vi "CH_LM App ResolutionMenu.vi"(4 "Action (query)":bool, 5 "error in":errorcluster, 6 "menubar":refnum<k9>, 7 "Menu String":string, 8 "Meter Index":i32) -> (0 "error out":errorcluster, 3 "Meter Index":i32)   [LabVIEW 2012, in "CH_LM App.lvlib"]
doc: "This VI is used to set/query the resolution of the displayed measurement value and check the corresponding menu items."
uses:
  CH_LM App.lvlib
  CH_LM.lvlib
  CH_LM/CH_LM Numeric Resolution.ctl
  CH_LM/CH_LM ProbeType.ctl
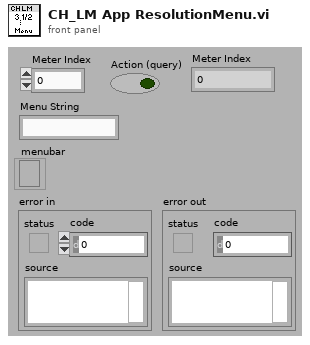
[diagram p1: front panel]
types:
  T1 = typedef "CH_LM.lvlib/CH_LM ProbeType.ctl" = enum16{"None", "Thermopile", "Pyroelectric", "Optical"}
  T2 = typedef "CH_LM.lvlib/CH_LM Numeric Resolution.ctl" = enum16{"3½", "4½", "5½", "6½"}
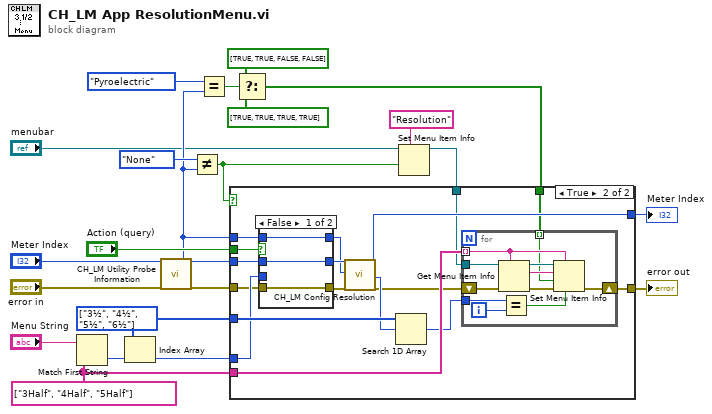
[diagram p0: block diagram]
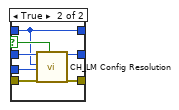
[diagram p3: hidden frame]
diagram:
  w22 = T2[] [enum."3½", enum."4½", enum."5½", enum."6½"] items=["3½", "4½", "5½", "6½"]
  w21 = string[] ["3Half", "4Half", "5Half"]
  n1 = Match First String(2:w21, 3:"Menu String") -> (0:w19:i32)  [unwired: 1 out]
  n2 = Index Array(array=w22, index=w19) -> (element=w20:T2)
  n3 = call "CH_LM Utility Probe Information.vi"("Meter Index"="Meter Index", "error in (no error)"="error in") -> ("Probe Type"=w8:T1, "Meter Index"=w15:i32, "error out"=w14:errorcluster)  [unwired: 15 out]
  n4 = Not Equal?(x=CH_LM_ProbeType."None" ("Probe Type"), y=w8) -> (x != y?=w1:bool)
  n5 = Equal?(x=CH_LM_ProbeType."Pyroelectric" ("Probe Type"), y=w8) -> (x = y?=w7:bool)
  n6 = Select(t=bool[] [TRUE, TRUE, FALSE, FALSE], s=w7, f=bool[] [TRUE, TRUE, TRUE, TRUE]) -> (s? t:f=w4:bool[])
  n7 = Set Menu Item Info(7:"Resolution" ("item tag"), 9:w1, 11:"menubar") -> (3:w2:refnum<k9>)  [unwired: 1 in, 4 out]
  n8 = case shown="True" w1 {
    tunnel: [w24 w42] -> w23
    tunnel: w22 -> [_ w41]
    tunnel: w21 -> [_ w40]
    tunnel: w20 -> [_ w38]
    tunnel: "Action (query)" -> [_ w37]
    tunnel: [w25 w34] -> w16
    tunnel: w15 -> [w25 w32]
    tunnel: w14 -> [w24 w31]
    tunnel: w8 -> [_ w29]
    tunnel: w4 -> [_ w28]
    tunnel: w2 -> [_ w27]
    frame False {
    }
    frame True {
      n9 = case shown="False" w37 {
        selector: w37 -> [_ w47]
        tunnel: [w44 w48] -> w35
        tunnel: [w45 w49] -> w36
        tunnel: w38 -> [_ w50]
        tunnel: w31 -> [w44 w51]
        tunnel: w32 -> [w45 w52]
        tunnel: w29 -> [w43 w46]
        tunnel: [w43 w46] -> w30
        frame False {
        }
        frame True {
          n10 = call "CH_LM Config Resolution.vi"("Meter Index"=w52, "Probe Type"=w46, "Resolution (3 1/2)"=w50, "error in (no error)"=w51, "Action (query)"=w47) -> ("Meter Index"=w49:i32, "error out"=w48:errorcluster)  [unwired: 13 out]
        }
      }
      n11 = call "CH_LM Config Resolution.vi"("Meter Index"=w36, "Probe Type"=w30, "error in (no error)"=w35) -> ("Meter Index"=w34:i32, "Resolution (3 1/2)"=w33:T2, "error out"=w26:errorcluster)  [unwired: 2 in, 12 out]
      n12 = Search 1D Array(1D array=w41, element=w33) -> (index of element=w39:i32)  [unwired: 1 out]
      n13 = for {
        tunnel: w27 -> [w60]
        shift-right: [w59] -> w42
        shift-left: w26 -> [w58]
        tunnel: w40 -> [w57] mode=indexing
        tunnel: w39 -> [w54]
        tunnel: w28 -> [w53] mode=indexing
        i -> [w56]
        n14 = Get Menu Item Info(7:w57, 8:w58, 11:w60) -> (0:w63:errorcluster, 2:w62:string, 3:w61:refnum<k9>)  [unwired: 4 out]
        n15 = Equal?(x=w54, y=w56) -> (x = y?=w55:bool)
        n16 = Set Menu Item Info(6:w55, 7:w57, 8:w63, 9:w53, 10:w62, 11:w61) -> (0:w59:errorcluster)  [unwired: 2 out]
      }
    }
  }
  "error out" <- w23
  "Meter Index" <- w16
